vi "Set Variant Property.vi"(6 "Control Ref Queue":T1, 8 "error in (no error)":errorcluster, 10 "Property In":variant, 11 "3D Surface.lvclass in":refnum<class "3D Surface.lvclass">) -> (0 "error out":errorcluster, 3 "3D Surface.lvclass":refnum<class "3D Surface.lvclass">)   [LabVIEW 2020, in "3D Surface.lvclass"]
uses:
  <vilib>/Math Plots/3D Math Plots/3D Surface/3D Surface/3D Surface.lvclass
  <vilib>/Math Plots/3D Math Plots/3D Surface/3D Surface/Typedef/3D Surface Property Array.ctl
  <vilib>/Math Plots/3D Math Plots/3D Surface/3D Surface/Typedef/3D Surface Property.ctl
  <vilib>/Math Plots/3D Math Plots/3D Plot/3D Plot/Typedef/Color Ramp Cluster.ctl
  <vilib>/Math Plots/3D Math Plots/3D Plot/3D Plot/Typedef/Line Type.ctl
  <vilib>/Math Plots/3D Math Plots/3D Plot/Action String/3DMathPlot Ctrl Act Queue.ctl
  <vilib>/Math Plots/3D Math Plots/3D Plot/Action String/3DMathPlot Ctrl Act Cluster.ctl
  <vilib>/Math Plots/3D Math Plots/3D Plot/Action String/3DMathPlot State Class.ctl
  <vilib>/Math Plots/3D Math Plots/3D Surface/3D Surface/3D Surface.lvclass/3D Surface.ctl
  <vilib>/Math Plots/3D Math Plots/3D Plot/3D Plot/3D Plot.lvclass
panel:
  in  "3D Surface Proprty Array":T2
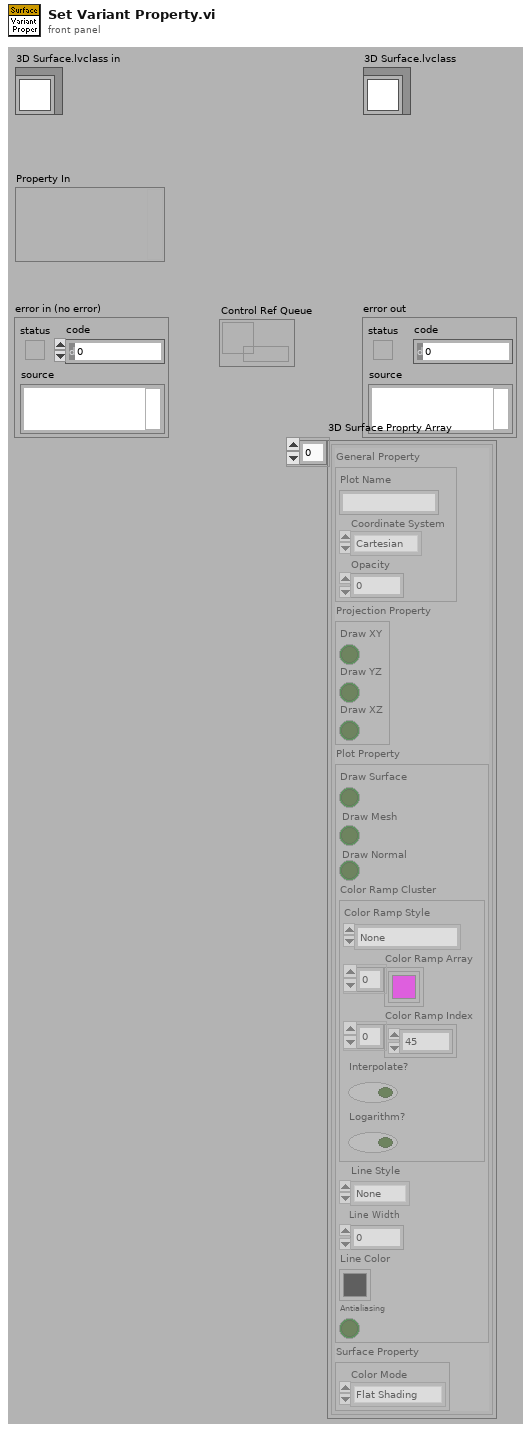
[diagram p1: front panel]
types:
  T1 = typedef "3DMathPlot Ctrl Act Queue.ctl" = refnum<queue>
  T2 = typedef "3D Surface.lvclass/3D Surface Property Array.ctl" = T3[]
  T3 = typedef "3D Surface.lvclass/3D Surface Property.ctl" = cluster{"General Property":cluster{"Plot Name":string, "Coordinate System":enum16{"Cartesian", "Cylindrical", "Spherical"}, "Opacity":sgl}, "Projection Property":cluster{"Draw XY":bool, "Draw YZ":bool, "Draw XZ":bool}, "Plot Property":cluster{"Draw Surface":bool, "Draw Mesh":bool, "Draw Normal":bool, "Color Ramp Cluster":T4, "Line Style":T5, "Line Width":sgl, "Line Color":u32, "Antialiasing":bool}, "Surface Property":cluster{"Color Mode":enum16{"Flat Shading", "Interpolated Shading"}}}
  T4 = typedef "3D Plot.lvclass/Color Ramp Cluster.ctl" = cluster{"Color Ramp Style":enum16{"None", "Shaded", "Color spectrum", "Grey scale", "Custom"}, "Color Ramp Array":u32[], "Color Ramp Index":i32[], "Interpolate?":bool, "Logarithm?":bool}
  T5 = typedef "3D Plot.lvclass/Line Type.ctl" = enum16{"None", "Solid", "Dash", "Dot", "Dash Dot"}
  T6 = typedef "3DMathPlot State Class.ctl" = enum16{"Update All Objects (Undo)", "Update Light Object Only", "Update Axis Object Only", "Update Plot Object Only", "Update Cursor Object Only", "Update Axis Plot Cursor Objects", "No Update"}
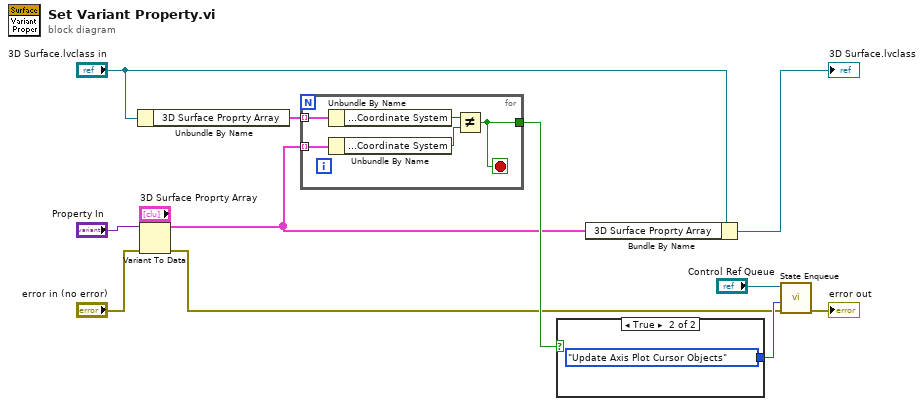
[diagram p0: block diagram]
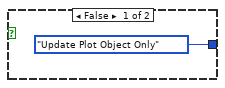
[diagram p2: hidden frame]
diagram:
  n1 = Unbundle By Name("3D Surface.lvclass in") -> ("3D Surface Proprty Array"=w9:T2)
  n2 = Variant To Data(error in="error in (no error)", type="3D Surface Proprty Array", Variant="Property In") -> (data=w5:T2, error out=w4:errorcluster)
  n3 = for {
    tunnel: w5 -> [w16] mode=indexing
    tunnel: w9 -> [w17] mode=indexing
    tunnel: [w13] -> w6
    stop <- w13 stop-if-true
    n4 = Unbundle By Name(w17) -> ("General Property.Coordinate System"=w15:enum16{"Cartesian", "Cylindrical", "Spherical"})
    n5 = Unbundle By Name(w16) -> ("General Property.Coordinate System"=w14:enum16{"Cartesian", "Cylindrical", "Spherical"})
    n6 = Not Equal?(x=w15, y=w14) -> (x != y?=w13:bool)
  }
  n7 = case shown="True" w6 {
    tunnel: [3DMathPlot_State_Class."Update Plot Object Only" ("Display State Change Class") 3DMathPlot_State_Class."Update Axis Plot Cursor Objects" ("Display State Change Class")] -> w8
    frame False {
    }
    frame True {
    }
  }
  n8 = Bundle By Name(cluster="3D Surface.lvclass in", "3D Surface Proprty Array"=w5) -> (→"3D Surface.lvclass":refnum<class "3D Surface.lvclass">)
  n9 = call <vilib>:"State Enqueue.vi"("error in (no error)"=w4, "Display State Change Class"=w8, "Control Ref Queue"="Control Ref Queue") -> ("error out"=→"error out":errorcluster)  [unwired: 8 out]
